vi "Initialize.vi"(8 "error in (no error)":errorcluster, 11 "File in":refnum<class "File.lvclass">) -> (0 "error out":errorcluster, 2 "File Path":path, 3 "File out":refnum<class "File.lvclass">)   [LabVIEW 2024, in "File.lvclass"]
uses:
  File.lvclass
  File.lvclass/File.ctl
  Read Include time.vi
  Read File format.vi
  Read Root Data Folder.vi
  Read Project folder .vi
  Read Index digits.vi
  Read File Prefix.vi
  Read File middle.vi
  Read Index file.vi
  Write Data File  Path.vi
  Write Settings File Path.vi
  Write Index  File Path.vi
  Write Index.vi
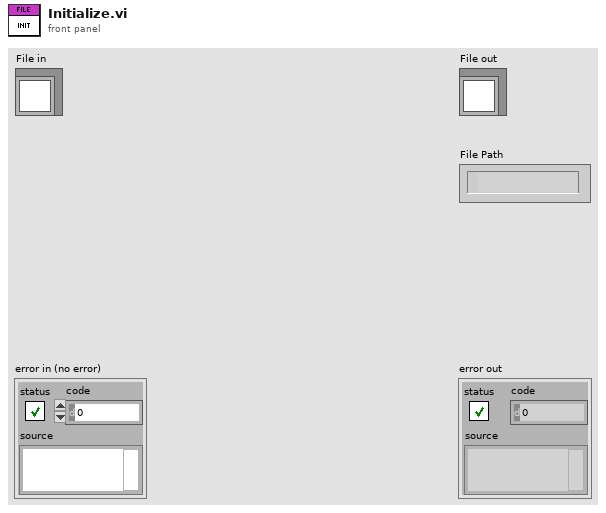
[diagram p1: front panel]
types:
  T1 = typedef "File formats.ctl" = enum16{"TDMS", "ASCII", "BINARY"}
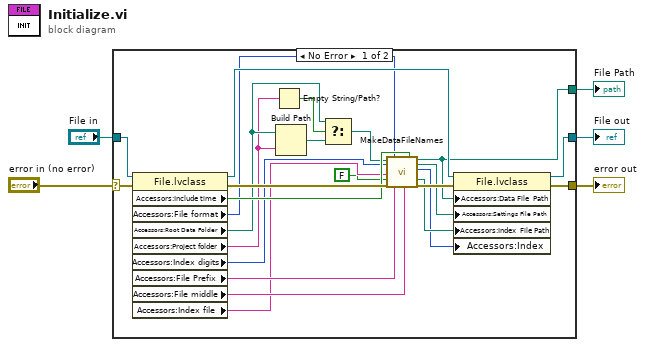
[diagram p0: block diagram]
diagram:
  n1 = case shown="No Error" "error in (no error)" {
    selector: "error in (no error)" -> [w28 w30]
    tunnel: [w22 w30] -> w2
    tunnel: [w21 w29] -> w3
    tunnel: "File in" -> [w25 w29]
    tunnel: [w20 _] -> w1
    frame No Error {
      n2 = property class="File.lvclass"(reference=w25, error in=w28) -> (reference out=w24:refnum<class "File.lvclass">, error out=w26:errorcluster, "Accessors:Include time"=w17:bool, "Accessors:File format"=w16:T1, "Accessors:Root Data Folder"=w13:path, "Accessors:Project folder "=w12:string, "Accessors:Index digits"=w15:i32, "Accessors:File Prefix"=w23:string, "Accessors:File middle"=w9:string, "Accessors:Index file"=w8:string)
      n3 = Empty String/Path?(string/path=w12) -> (empty?=w14:bool)
      n4 = Build Path(base path=w13, name or relative path=w12) -> (appended path=w11:path)
      n5 = Select(t=w13, s=w14, f=w11) -> (s? t:f=w10:path)
      n6 = call "MakeDataFileNames.vi"("Root Data Folder"=w10, "Index digits"=w15, "Index file"=w8, "Interactive"=FALSE, "Error In"=w26, "File format"=w16, "File Prefix"=w23, "File middle"=w9, "Include time"=w17) -> ("Data File  Path"=w20:path, "Settings File Path"=w19:path, "Index out"=w6:i32, "Index  File Path"=w18:path, "Error Out"=w27:errorcluster)  [unwired: 5 in, 1 out]
      n7 = property class="File.lvclass"(reference=w24, error in=w27, "Accessors:Data File  Path"=w20, "Accessors:Settings File Path"=w19, "Accessors:Index  File Path"=w18, "Accessors:Index"=w6) -> (reference out=w21:refnum<class "File.lvclass">, error out=w22:errorcluster)
    }
    frame Error {
    }
  }
  "error out" <- w2
  "File out" <- w3
  "File Path" <- w1
